vi "Demo - Simple Use Testing.vi"() -> ()   [LabVIEW 2013]
uses:
  Get Variable/Scalar - String.vi
  Get Variable/Scalar - Real.vi
  Get Variable/Scalar - Complex.vi
  Get Variable/Vector - Reals.vi
  Get Variable/Vector - Strings.vi
  Get Variable/Vector - Complex.vi
  GOLPI library.lvlib
panel:
  in  "data type array 3":cdb[](array[numeric])
  in  "data type array 2":string[](array[string])
  in  "data type 4":cdb
  in  "data type 3":dbl
  in  "Get variable":T1(tab)=enum."vector strings"
  out "value":string
  out "value 3":dbl format="%.2f"
  out "value 4":cdb format="%.2f"
  out "size(s) 2":i32
  out "vector 2":string[](array[string])
  out "vector":dbl[](array[numeric])
  out "size(s)":i32
  out "size(s) 3":i32
  out "vector 3":cdb[](array[numeric])
  in  "data type array":dbl[](array[numeric])
  in  "data type":string
  in  "variable name":string="x"
  in  "command":string="x=[1 2 3]\ndisp('OK')"
  out "GNU Octave version":string
  out "exit code":i32
  out "error out":errorcluster
  out "read buffer":string
  in  "Octave binary directory":path=path "C:/Program Files/Octave-3.6.2/bin"
  in  "Working directory":path=path "C:/"
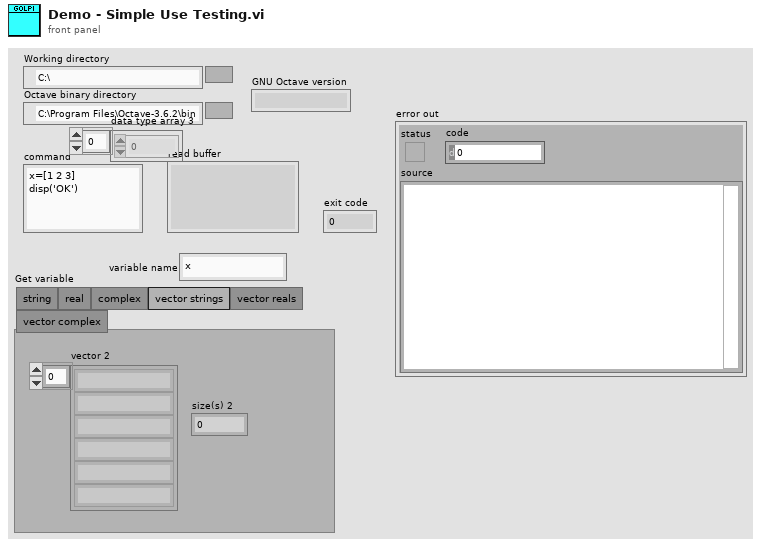
[diagram p1: front panel]
types:
  T1 = enum32{"string", "real", "complex", "vector strings", "vector reals", "vector complex"}
  T2 = typedef "LV Process.lvlibp/Pipe Handle.ctl" = cluster{"lv_proc.dll file path":path, "process instance handle":u32[]}
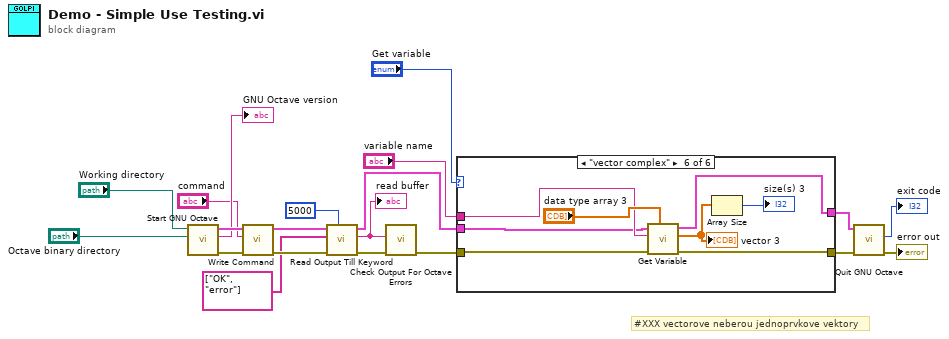
[diagram p0: block diagram]
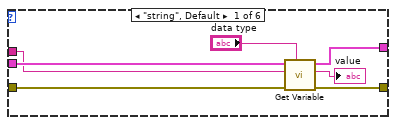
[diagram p2: hidden frame]
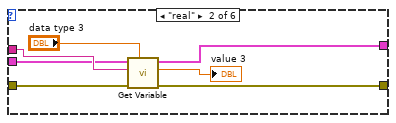
[diagram p3: hidden frame]
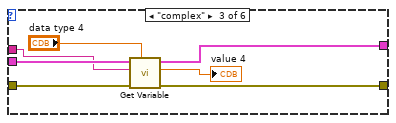
[diagram p4: hidden frame]
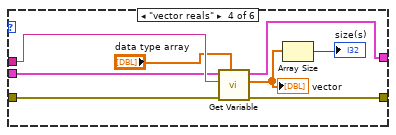
[diagram p5: hidden frame]
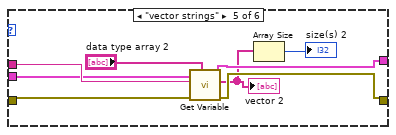
[diagram p6: hidden frame]
diagram:
  # "#XXX vectorove neberou jednoprvkove vektory"
  n1 = call "Start GNU Octave.vi"("Octave binary directory"="Octave binary directory", "Working directory"="Working directory") -> ("error out"=w16:errorcluster, "GNU Octave version"=→"GNU Octave version":string, "pipe out"=w18:T2)  [unwired: 6 in, 1 out]
  n2 = call "Write Command.vi"("error in"=w16, "command"="command", "pipe in"=w18) -> ("error out"=w15:errorcluster, "pipe out"=w17:T2)  [unwired: 7 in]
  n3 = call "Read Output Till Keyword.vi"("timeout [ms]"=u32 5000, "error in"=w15, "keywords"=string[] ["OK", "error"], "pipe in"=w17) -> ("error out"=w7:errorcluster, "read buffer"=w5:string, "pipe out"=w11:T2)  [unwired: 4 in, 1 out]
  "read buffer" <- w5
  n4 = call "Check Output For Octave Errors.vi"("error in"=w7, "read buffer"=w5) -> ("error out"=w6:errorcluster)  [unwired: 9 in]
  n5 = case shown="\"vector complex\"" "Get variable" {
    tunnel: w11 -> [w26 w31 w39 w47 w54 w61]
    tunnel: [w23 w29 w36 w46 w51 w58] -> w10
    tunnel: [w24 w28 w35 w45 w52 w59] -> w9
    tunnel: "variable name" -> [w21 w32 w37 w48 w55 w62]
    tunnel: w6 -> [w25 w33 w38 w49 w53 w60]
    frame "string", Default {
      n6 = call-poly "Get Variable.vi"("data type of variable"="data type", "error in"=w25, "variable name"=w21, "pipe in"=w26) -> ("error out"=w24:errorcluster, "value"=→"value":string, "pipe out"=w23:T2)  [unwired: 5 in]
    }
    frame "real" {
      n7 = call-poly "Get Variable.vi"("data type of variable"="data type 3", "error in"=w33, "variable name"=w32, "pipe in"=w31) -> ("error out"=w28:errorcluster, "value"=→"value 3":dbl, "pipe out"=w29:T2)  [unwired: 5 in]
    }
    frame "complex" {
      n8 = call-poly "Get Variable.vi"("data type of variable"="data type 4", "error in"=w38, "variable name"=w37, "pipe in"=w39) -> ("error out"=w35:errorcluster, "value"=→"value 4":cdb, "pipe out"=w36:T2)  [unwired: 5 in]
    }
    frame "vector reals" {
      n9 = call-poly "Get Variable.vi"("data type of variable"="data type array", "error in"=w49, "variable name"=w48, "pipe in"=w47) -> ("error out"=w45:errorcluster, "value"=w42:dbl[], "pipe out"=w46:T2)  [unwired: 5 in]
      "vector" <- w42
      n10 = Array Size(array=w42) -> (size(s)=→"size(s)":i32)
    }
    frame "vector strings" {
      n11 = call-poly "Get Variable.vi"("data type of variable"="data type array 2", "error in"=w53, "variable name"=w55, "pipe in"=w54) -> ("error out"=w52:errorcluster, "value"=w50:string[], "pipe out"=w51:T2)  [unwired: 5 in]
      "vector 2" <- w50
      n12 = Array Size(array=w50) -> (size(s)=→"size(s) 2":i32)
    }
    frame "vector complex" {
      n13 = call-poly "Get Variable.vi"("data type of variable"="data type array 3", "error in"=w60, "variable name"=w62, "pipe in"=w61) -> ("error out"=w59:errorcluster, "value"=w63:cdb[], "pipe out"=w58:T2)  [unwired: 5 in]
      "vector 3" <- w63
      n14 = Array Size(array=w63) -> (size(s)=→"size(s) 3":i32)
    }
  }
  n15 = call "Quit GNU Octave.vi"("error in"=w9, "pipe in"=w10) -> ("error out"=→"error out":errorcluster, "exit code"=→"exit code":i32)  [unwired: 8 in]
